vi "Constructor.vi"(8 "error in (no error)":errorcluster, 11 "Michell Easydew in":refnum<class "Michell Easidew.lvclass">) -> (0 "error out":errorcluster, 3 "Michell Easydew out":refnum<class "Michell Easidew.lvclass">)   [LabVIEW 2011, in "Michell Easidew.lvclass"]
uses:
  Michell Easidew.lvclass
  Dew Point Scale.ctl
  Michell Easidew.lvclass/Michell Easidew.ctl
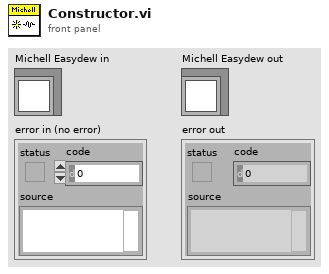
[diagram p1: front panel]
types:
  T1 = typedef "Michell Easidew.lvclass/Dew Point Scale.ctl" = enum16{"Celcius", "Fahrenheit"}
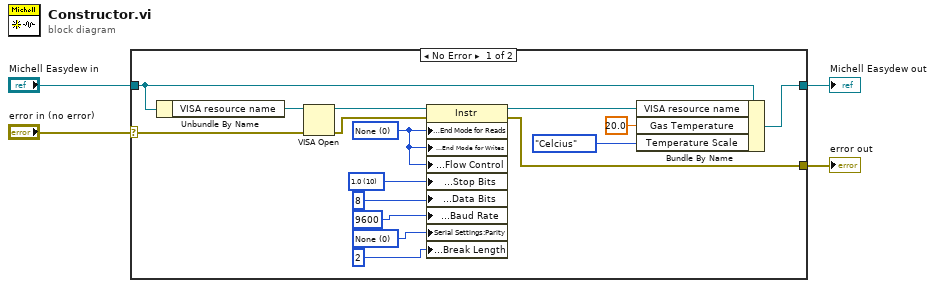
[diagram p0: block diagram]
diagram:
  n1 = case shown="No Error" "error in (no error)" {
    selector: "error in (no error)" -> [w8 w22]
    tunnel: [w7 w22] -> w3
    tunnel: [w9 w21] -> w1
    tunnel: "Michell Easydew in" -> [w11 w21]
    frame No Error {
      w15 = u16 0 items=["None", "Odd", "Even", "Mark", "Space"] ("Serial Settings:Parity")
      w18 = u16 10 items=["1.0"=10, "1.5"=15, "2.0"=20] ("Serial Settings:Serial Stop Bits")
      w19 = u16 0 items=["None", "Last Bit", "TermChar"] ("Serial Settings:End Mode for Reads")
      n2 = Unbundle By Name(w11) -> ("VISA resource name"=w12:refnum<visa-resource-name>)
      n3 = VISA Open(error in (no error)=w8, VISA resource name=w12) -> (VISA resource name=w20:refnum<visa-resource-name>, error out=w13:errorcluster)  [unwired: 3 in]
      n4 = property class="Instr"(reference=w20, error in=w13, "Serial Settings:End Mode for Reads"=w19, "Serial Settings:End Mode for Writes"=w19, "Serial Settings:Flow Control"=w19, "Serial Settings:Stop Bits"=w18, "Serial Settings:Data Bits"=u16 8 ("Serial Settings:Serial Data Bits"), "Serial Settings:Baud Rate"=u32 9600, "Serial Settings:Parity"=w15, "Serial Settings:Break Length"=i16 2) -> (reference out=w10:refnum<visa-resource-name>, error out=w7:errorcluster)
      n5 = Bundle By Name(cluster=w11, "VISA resource name"=w10, "Gas Temperature"=20.0, "Temperature Scale"=Dew_Point_Scale."Celcius") -> (w9:refnum<class "Michell Easidew.lvclass">)
    }
    frame Error {
    }
  }
  "error out" <- w3
  "Michell Easydew out" <- w1
